vi "Constants.vi"() -> ()   [LabVIEW 2020, in "ARINC 429 Scripting.lvlib"]
doc: "Use this Global VI to access the GUIDs assigned to the page resources of the Custom Device."
uses:
  ARINC 429 Scripting.lvlib
panel:
  in  "Prop.Transfer.Speed":string="TransferSpeed"
  in  "SDI":string="SDI"
  in  "SSM":string="SSM"
  in  "Parity":string="Parity"
  in  "Prop.Port":string="Port"
  in  "Prop.Word.Initial.Raw.Value":string="WordInitialRawValue"
  in  "Prop.Label":string="Label"
  in  "Prop.Raw.Data.Bits":string="RawData Bits"
  in  "Prop.SDI.Enabled":string="SDI_Enabled"
  in  "Prop.SDI.Value":string="SDIValue"
  in  "Prop.TxRate":string="txRate"
  in  "Prop.Transfer.Type":string="TransferType"
  in  "Prop.Default.word":string="Default word"
  in  "Prop.Encoding.Type":string="Encoding Type"
  in  "Prop.Start.Bit":string="Start Bit"
  in  "Prop.Num.Bits":string="Num Bits"
  in  "Prop.Signed?":string="Signed?"
  in  "Prop.Scale.Fac":string="ScaleFac"
  in  "Prop.Scale.Offset":string="ScaleOffset"
  in  "Prop.Unit":string="Unit"
  in  "Prop.Baud.Rate":string="Baud.Rate"
  in  "Prop.Database.Path":string="Database.Path"
  in  "Prop.Database.Name":string="Database.Name"
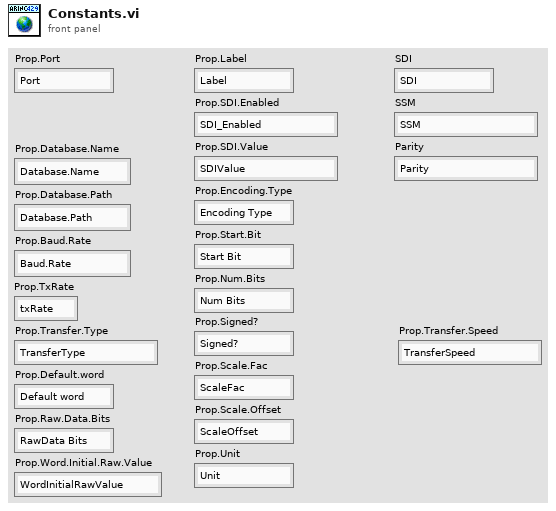
[diagram p1: front panel]
diagram:
